vi "Autonomous Independent.vi"   [LabVIEW 2011]
doc: "This VI is called when autonomous begins, and will automatically be terminated when autonomous ends. You can carry out timed or sensor driven robot movement independently without needing to return to the caller."
uses:
  Robot Global Data.vi
  <vilib>/Rock Robotics/WPI/RobotDrive/WPI_RobotDriveArcadeDrive_Standard(NoSaturation).vi
types:
  T1 = typedef "WPI_JoystickDevRef.ctl" = cluster{"Device":T2}
  T2 = typedef "WPI_JoystickDeviceEnum.ctl" = enum16{"USB 1", "USB 2", "USB 3", "USB 4", "Kinect 1", "Kinect 2"}
  T3 = cluster{"axis 1 (x)":dbl, "axis 2 (y)":dbl, "axis 3 (throttle)":dbl, "axis 4":dbl, "axis 5":dbl, "axis 6":dbl}
  T4 = typedef "WPI_RobotDriveDevRef.ctl" = cluster{"DevStatus":errorcluster, "Motors[]":T5[], "Square Inputs":bool, "Max Output":dbl, "Isochronous":bool}
  T5 = typedef "WPI_MotorControlDeviceRef.ctl" = cluster{"DeviceStatus":errorcluster, "Type":enum16{"PWM", "CAN"}, "PWM":cluster{"Digital Module":T6, "PWM Channel":T7, "DeadBand":T8}, "CAN":cluster{"Device Number":u8, "Control Mode":T9, "Semaphore":T10, "Max Vout":dbl}, "Invert":bool, "TransformRef":T11, "InvTransformRef":T11}
  T6 = typedef "FPGA_TypedefDigitalModule.ctl" = enum16{"Digital Module 1", "Digital Module 2"}
  T7 = typedef "FPGA_DIOPWMChannel.ctl" = enum8{"PWM 1", "PWM 2", "PWM 3", "PWM 4", "PWM 5", "PWM 6", "PWM 7", "PWM 8", "PWM 9", "PWM 10", "Invalid"}
  T8 = typedef "WPI_PWMDeadband.ctl" = cluster{"Name":string, "maxPositivePwm":i32, "minPositivePwm":i32, "centerPwm":i32, "maxNegativePwm":i32, "minNegativePwm":i32, "angularRange":u16}
  T9 = typedef "WPI_CANJaguar_ControlMode.ctl" = enum8{"Percent VBus", "Current", "Speed", "Position", "Voltage"}
  T10 = typedef "Semaphore RefNum" = refnum<k1>
  T11 = typedef "WPI_PWMTransform_ConPane.ctl" = refnum<vi>
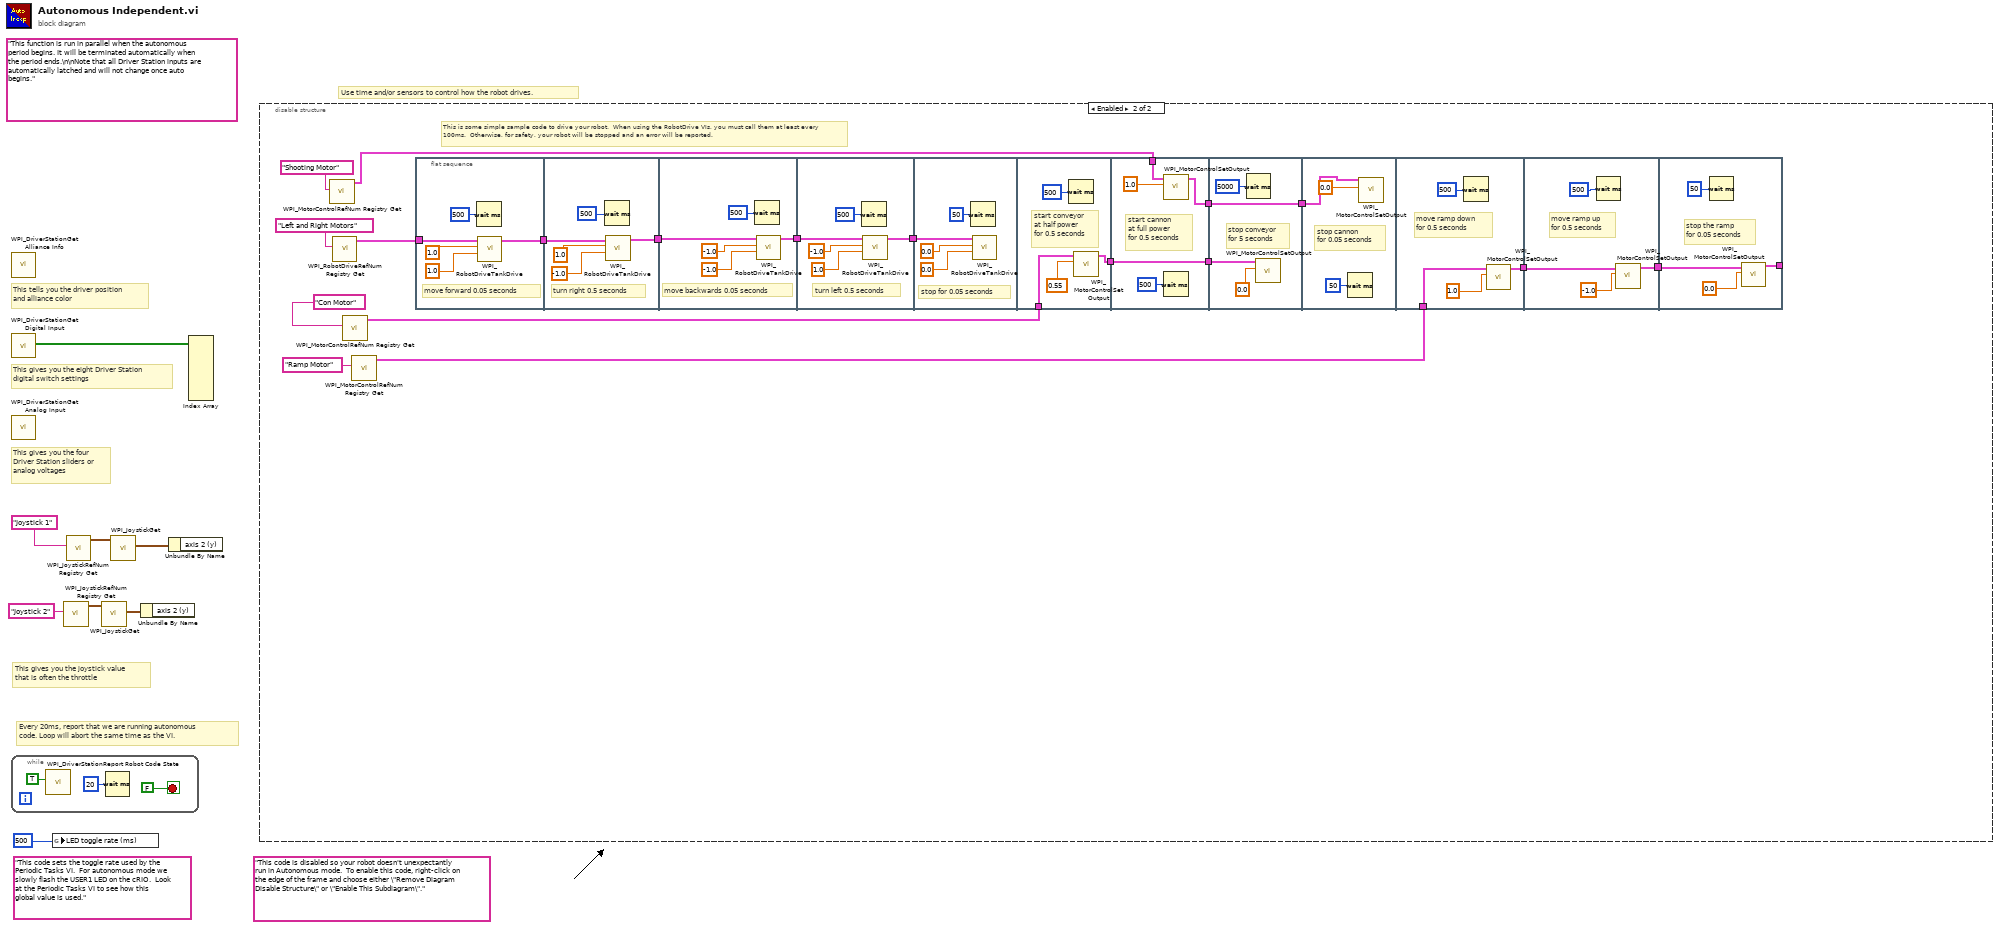
[diagram p0: block diagram]
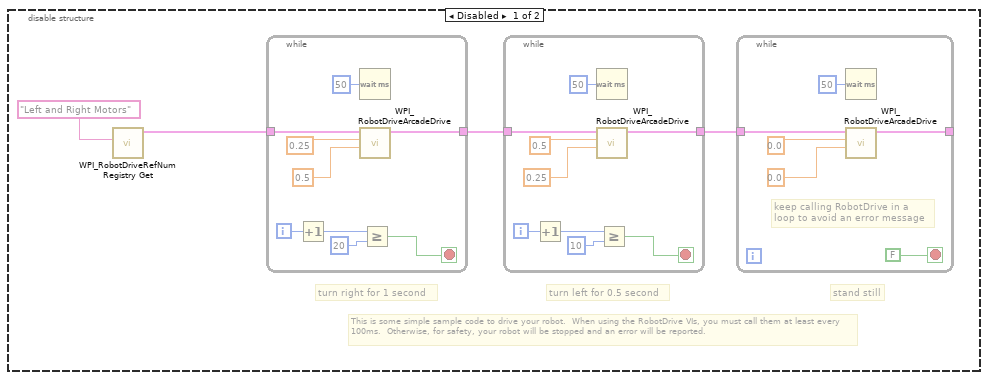
[diagram p2: hidden frame]
diagram:
  (unwired) "This code sets the toggle rate used by the Periodic Tasks VI.  For autonomous mode we slowly flash the USER1 LED on the cRIO.  Look at the Periodic Tasks VI to see how this global value is used."
  (unwired) "This code is disabled so your robot doesn't unexpectantly run in Autonomous mode.  To enable this code, right-click on the edge of the frame and choose either \"Remove Diagram Disable Structure\" or \"Enable This Subdiagram\"."
  (unwired) "This function is run in parallel when the autonomous period begins. It will be terminated automatically when the period ends.\n\nNote that all Driver Station inputs are automatically latched and will not change once auto begins."
  # "Every 20ms, report that we are running autonomous\ncode. Loop will abort the same time as the VI."
  # "This gives you the joystick value\nthat is often the throttle"
  # "Use time and/or sensors to control how the robot drives."
  # "This tells you the driver position\nand alliance color"
  # "This gives you the eight Driver Station\ndigital switch settings"
  # "This gives you the four\nDriver Station sliders or\nanalog voltages"
  n1 = call <vilib>:"WPI_DriverStationGet Alliance Info.vi"() -> ()  [unwired: 12 out]
  n2 = call <vilib>:"WPI_DriverStationGet Digital Input.vi"() -> ("Driver Station Digital Input (1-8)"=w8:bool[])  [unwired: 11 out]
  n3 = call <vilib>:"WPI_DriverStationGet Analog Input.vi"() -> ()  [unwired: 12 out]
  n4 = while {
    stop <- FALSE stop-if-true
    n5 = call <vilib>:"WPI_DriverStationReport Robot Code State.vi"("Autonomous"=TRUE) -> ()  [unwired: 10 in, 1 out]
    n6 = Wait (ms)(milliseconds to wait=u32 20) -> ()  [unwired: 1 out]
  }
  n7 = global write "Robot Global Data.vi" "LED toggle rate (ms)"(u32 500 ("LED ms toggle rate")) -> ()
  n8 = call <vilib>:"WPI_JoystickRefNum Registry Get.vi"("refnum name"="Joystick 2") -> ("JoystickDevRef"=w1:T1)  [unwired: 1 in, 9 out]
  n9 = call <vilib>:"WPI_JoystickRefNum Registry Get.vi"("refnum name"="Joystick 1") -> ("JoystickDevRef"=w5:T1)  [unwired: 1 in, 9 out]
  n10 = call <vilib>:"WPI_JoystickGet.vi"("JoystickDevRef"=w1) -> ("Axes"=w3:T3)  [unwired: 1 in, 5 out]
  n11 = call <vilib>:"WPI_JoystickGet.vi"("JoystickDevRef"=w5) -> ("Axes"=w6:T3)  [unwired: 1 in, 5 out]
  n12 = Unbundle By Name(w3) -> ()  [unwired: 1 out]
  n13 = Unbundle By Name(w6) -> ()  [unwired: 1 out]
  n14 = Index Array(array=w8) -> ()  [unwired: 8 in, 8 out]
  n15 = disable-structure shown="Enabled" {
    frame Disabled {
      # "This is some simple sample code to drive your robot.  When using the RobotDrive VIs, you must call them at least every 100ms.  Otherwise, for safety, your robot will be stopped and an error will be reported."
      # "stand still"
      # "turn left for 0.5 second"
      # "turn right for 1 second"
      n16 = call <vilib>:"WPI_RobotDriveRefNum Registry Get.vi"("refnum name"="Left and Right Motors") -> ("RobotDriveDevRef"=w14:T4)  [unwired: 1 in, 9 out]
      n17 = while {
        tunnel: w14 -> [w39]
        tunnel: [w32] -> w13
        i -> [w35]
        stop <- w33 stop-if-true
        n18 = Increment(x=w35) -> (x+1=w31:i32)
        n19 = Wait (ms)(milliseconds to wait=u32 50) -> ()  [unwired: 1 out]
        n20 = call-poly <vilib>:"WPI_RobotDriveArcadeDrive.vi"("Y axis value"=0.5 ("X axis value"), "X axis value"=0.25, "RobotDriveDevRef"=w39) -> ("RobotDriveDevRef"=w32:T4)  [unwired: 1 in, 7 out]
        n21 = Greater Or Equal?(x=w31, y=20) -> (x >= y?=w33:bool)
      }
      n22 = while {
        tunnel: w13 -> [w30]
        tunnel: [w23] -> w12
        i -> [w26]
        stop <- w24 stop-if-true
        n23 = Increment(x=w26) -> (x+1=w22:i32)
        n24 = Wait (ms)(milliseconds to wait=u32 50) -> ()  [unwired: 1 out]
        n25 = call-poly <vilib>:"WPI_RobotDriveArcadeDrive.vi"("Y axis value"=0.25 ("X axis value"), "X axis value"=0.5, "RobotDriveDevRef"=w30) -> ("RobotDriveDevRef"=w23:T4)  [unwired: 1 in, 7 out]
        n26 = Greater Or Equal?(x=w22, y=10) -> (x >= y?=w24:bool)
      }
      n27 = while {
        tunnel: w12 -> [w21]
        tunnel: [w17] -> _
        stop <- FALSE stop-if-true
        # "keep calling RobotDrive in a loop to avoid an error message"
        n28 = Wait (ms)(milliseconds to wait=u32 50) -> ()  [unwired: 1 out]
        n29 = call-poly <vilib>:"WPI_RobotDriveArcadeDrive.vi"("Y axis value"=0.0 ("X axis value"), "X axis value"=0.0, "RobotDriveDevRef"=w21) -> ("RobotDriveDevRef"=w17:T4)  [unwired: 1 in, 7 out]
      }
    }
    frame Enabled {
      # "This is some simple sample code to drive your robot.  When using the RobotDrive VIs, you must call them at least every 100ms.  Otherwise, for safety, your robot will be stopped and an error will be reported."
      n30 = call <vilib>:"WPI_MotorControlRefNum Registry Get.vi"("refnum name"="Shooting Motor") -> ("MotorControlDevRef"=w49:T5)  [unwired: 9 in, 1 out]
      n31 = call <vilib>:"WPI_RobotDriveRefNum Registry Get.vi"("refnum name"="Left and Right Motors") -> ("RobotDriveDevRef"=w54:T4)  [unwired: 1 in, 9 out]
      n32 = call <vilib>:"WPI_MotorControlRefNum Registry Get.vi"("refnum name"="Con Motor") -> ("MotorControlDevRef"=w50:T5)  [unwired: 9 in, 1 out]
      n33 = call <vilib>:"WPI_MotorControlRefNum Registry Get.vi"("refnum name"="Ramp Motor") -> ("MotorControlDevRef"=w42:T5)  [unwired: 9 in, 1 out]
      n34 = flat-sequence {
        tunnel: w54 -> [w59]
        tunnel: [w58] -> w56
        tunnel: w56 -> [w64]
        tunnel: [w63] -> w55
        tunnel: w55 -> [w69]
        tunnel: [w68] -> w53
        tunnel: w53 -> [w74]
        tunnel: [w73] -> w44
        tunnel: w44 -> [w78]
        tunnel: w50 -> [w84]
        tunnel: [w83] -> w47
        tunnel: w49 -> [w89]
        tunnel: [w88] -> w48
        tunnel: w47 -> [w88]
        tunnel: [w87] -> w45
        tunnel: w48 -> [w92]
        tunnel: [w91] -> w46
        tunnel: w45 -> [w91]
        tunnel: w46 -> [w95]
        tunnel: w42 -> [w99]
        tunnel: [w98] -> w41
        tunnel: w41 -> [w103]
        tunnel: [w102] -> w40
        tunnel: w40 -> [w107]
        tunnel: [w106] -> _
        frame #0 {
          # "move forward 0.05 seconds"
          n35 = Wait (ms)(milliseconds to wait=u32 500) -> ()  [unwired: 1 out]
          n36 = call <vilib>:"WPI_RobotDriveTankDrive.vi"("Right axis value"=1.0 ("X axis value"), "Left axis value"=1.0 ("X axis value"), "RobotDriveDevRef"=w59) -> ("RobotDriveDevRef"=w58:T4)  [unwired: 7 in, 1 out]
        }
        frame #1 {
          # "turn right 0.5 seconds"
          n37 = Wait (ms)(milliseconds to wait=u32 500) -> ()  [unwired: 1 out]
          n38 = call <vilib>:"WPI_RobotDriveTankDrive.vi"("Right axis value"=-1.0 ("X axis value"), "Left axis value"=1.0 ("X axis value"), "RobotDriveDevRef"=w64) -> ("RobotDriveDevRef"=w63:T4)  [unwired: 7 in, 1 out]
        }
        frame #2 {
          # "move backwards 0.05 seconds"
          n39 = Wait (ms)(milliseconds to wait=u32 500) -> ()  [unwired: 1 out]
          n40 = call <vilib>:"WPI_RobotDriveTankDrive.vi"("Right axis value"=-1.0 ("X axis value"), "Left axis value"=-1.0 ("X axis value"), "RobotDriveDevRef"=w69) -> ("RobotDriveDevRef"=w68:T4)  [unwired: 7 in, 1 out]
        }
        frame #3 {
          # "turn left 0.5 seconds"
          n41 = Wait (ms)(milliseconds to wait=u32 500) -> ()  [unwired: 1 out]
          n42 = call <vilib>:"WPI_RobotDriveTankDrive.vi"("Right axis value"=1.0 ("X axis value"), "Left axis value"=-1.0 ("X axis value"), "RobotDriveDevRef"=w74) -> ("RobotDriveDevRef"=w73:T4)  [unwired: 7 in, 1 out]
        }
        frame #4 {
          # "stop for 0.05 seconds"
          n43 = Wait (ms)(milliseconds to wait=u32 50) -> ()  [unwired: 1 out]
          n44 = call <vilib>:"WPI_RobotDriveTankDrive.vi"("Right axis value"=0.0 ("X axis value"), "Left axis value"=0.0 ("X axis value"), "RobotDriveDevRef"=w78) -> ()  [unwired: 7 in, 2 out]
        }
        frame #5 {
          # "start conveyor\nat half power\nfor 0.5 seconds"
          n45 = Wait (ms)(milliseconds to wait=u32 500) -> ()  [unwired: 1 out]
          n46 = call <vilib>:"WPI_MotorControlSetOutput.vi"("Output"=0.55 ("X axis value"), "MotorControlDevRef"=w84) -> ("MotorControlDevRef"=w83:T5)  [unwired: 8 in, 1 out]
        }
        frame #6 {
          # "start cannon\nat full power\nfor 0.5 seconds"
          n47 = call <vilib>:"WPI_MotorControlSetOutput.vi"("Output"=1.0 ("X axis value"), "MotorControlDevRef"=w89) -> ("MotorControlDevRef"=w87:T5)  [unwired: 8 in, 1 out]
          n48 = Wait (ms)(milliseconds to wait=u32 500) -> ()  [unwired: 1 out]
        }
        frame #7 {
          # "stop conveyor\nfor 5 seconds"
          n49 = Wait (ms)(milliseconds to wait=u32 5000) -> ()  [unwired: 1 out]
          n50 = call <vilib>:"WPI_MotorControlSetOutput.vi"("Output"=0.0 ("X axis value"), "MotorControlDevRef"=w92) -> ()  [unwired: 8 in, 2 out]
        }
        frame #8 {
          # "stop cannon\nfor 0.05 seconds"
          n51 = Wait (ms)(milliseconds to wait=u32 50) -> ()  [unwired: 1 out]
          n52 = call <vilib>:"WPI_MotorControlSetOutput.vi"("Output"=0.0 ("X axis value"), "MotorControlDevRef"=w95) -> ()  [unwired: 8 in, 2 out]
        }
        frame #9 {
          # "move ramp down\nfor 0.5 seconds"
          n53 = Wait (ms)(milliseconds to wait=u32 500) -> ()  [unwired: 1 out]
          n54 = call <vilib>:"WPI_MotorControlSetOutput.vi"("Output"=1.0, "MotorControlDevRef"=w99) -> ("MotorControlDevRef"=w98:T5)  [unwired: 8 in, 1 out]
        }
        frame #10 {
          # "move ramp up\nfor 0.5 seconds"
          n55 = Wait (ms)(milliseconds to wait=u32 500) -> ()  [unwired: 1 out]
          n56 = call <vilib>:"WPI_MotorControlSetOutput.vi"("Output"=-1.0, "MotorControlDevRef"=w103) -> ("MotorControlDevRef"=w102:T5)  [unwired: 8 in, 1 out]
        }
        frame #11 {
          # "stop the ramp\nfor 0.05 seconds"
          n57 = Wait (ms)(milliseconds to wait=u32 50) -> ()  [unwired: 1 out]
          n58 = call <vilib>:"WPI_MotorControlSetOutput.vi"("Output"=0.0, "MotorControlDevRef"=w107) -> ("MotorControlDevRef"=w106:T5)  [unwired: 8 in, 1 out]
        }
      }
    }
  }
